vi "Format Target Name.vi"(8 "error in":errorcluster, 11 "OD Entry in":refnum<class "OD Entry.lvclass">) -> (0 "error out":errorcluster, 2 "Name":string, 3 "OD Entry out":refnum<class "OD Entry.lvclass">)   [LabVIEW 2019, in "PDO Grid.lvlib" / "PDO Mapping.lvclass"]
uses:
  PDO Mapping.lvclass
  Core/OD Entry/OD Entry.lvclass
  Core/OD Sub-Entry/OD Sub-Entry.lvclass
  D:/git/EDS-File-Viewer/source/Core/OD Entry/OD Entry.lvclass
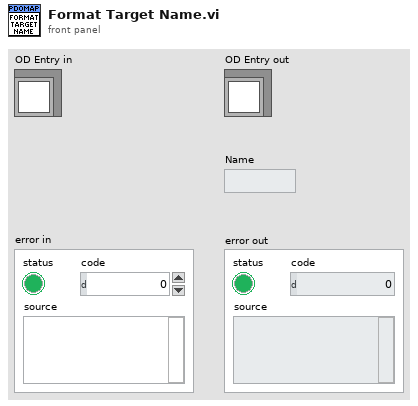
[diagram p1: front panel]
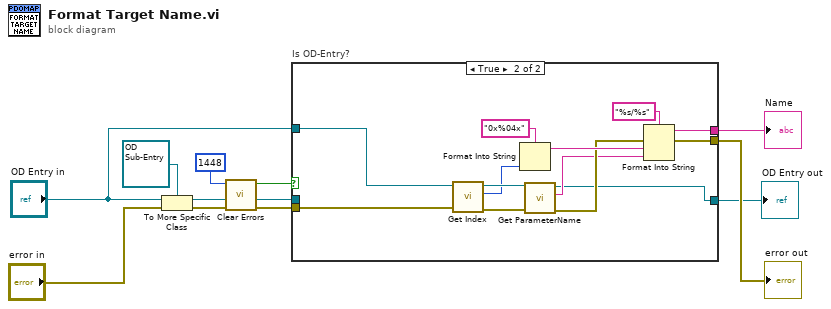
[diagram p0: block diagram]
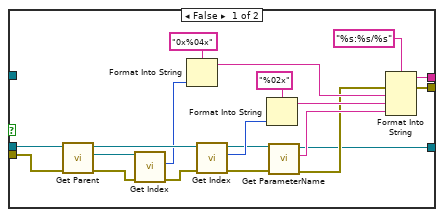
[diagram p2: hidden frame]
diagram:
  n1 = To More Specific Class(target class=refnum<class "OD Sub-Entry.lvclass"> refnum ("Electronic Datasheet.lvlib:OD Sub-Entry"), reference="OD Entry in", error in="error in") -> (specific class reference=w6:refnum<class "OD Sub-Entry.lvclass">, error out=w7:errorcluster)
  n2 = call <vilib>:"Clear Errors.vi"("error in (no error)"=w7, "specific error code to clear (0: all)"=1448) -> ("error out"=w4:errorcluster, "specific error cleared?"=w3:bool)  [unwired: 4 in]
  n3 = case "Is OD-Entry?" shown="True" w3 {
    tunnel: [w21 w33] -> w11
    tunnel: [w19 w35] -> w10
    tunnel: [w18 w34] -> w8
    tunnel: w6 -> [w12 _]
    tunnel: w4 -> [w17 w38]
    tunnel: "OD Entry in" -> [_ w32]
    frame False {
      n4 = call "Get Parent.vi"("Error In"=w17, "reference in"=w12) -> ("Error Out"=w16:errorcluster, "Parent"=w15:refnum<class "OD Entry.lvclass">, "reference out"=w31:refnum<class "OD Sub-Entry.lvclass">)  [unwired: 7 in]
      n5 = call "Get Index.vi"("Error In"=w16, "reference in"=w15) -> ("Error Out"=w30:errorcluster, "Index"=w13:u16)  [unwired: 7 in, 1 out]
      n6 = Format Into String(format string="0x%04x", w13) -> (resulting string=w24:string)  [unwired: 2 in, 1 out]
      n7 = call "Get Index.vi"("Error In"=w30, "reference in"=w31) -> ("Error Out"=w26:errorcluster, "Index"=w28:u16, "reference out"=w27:refnum<class "OD Sub-Entry.lvclass">)  [unwired: 7 in]
      n8 = Format Into String(format string="%02x", w28) -> (resulting string=w23:string)  [unwired: 2 in, 1 out]
      n9 = call "Get ParameterName.vi"("Error In"=w26, "reference in"=w27) -> ("Error Out"=w20:errorcluster, "ParameterName"=w22:string, "reference out"=w18:refnum<class "OD Sub-Entry.lvclass">)  [unwired: 7 in]
      n10 = Format Into String(format string="%s:%s/%s", error in=w20, w24, w23, w22) -> (resulting string=w21:string, error out=w19:errorcluster)  [unwired: 1 in]
    }
    frame True {
      n11 = call "Get Index.vi"("Error In"=w38, "reference in"=w32) -> ("Error Out"=w43:errorcluster, "Index"=w37:u16, "reference out"=w44:refnum<class "OD Entry.lvclass">)  [unwired: 7 in]
      n12 = Format Into String(format string="0x%04x", w37) -> (resulting string=w41:string)  [unwired: 2 in, 1 out]
      n13 = call "Get ParameterName.vi"("Error In"=w43, "reference in"=w44) -> ("Error Out"=w40:errorcluster, "ParameterName"=w36:string, "reference out"=w34:refnum<class "OD Entry.lvclass">)  [unwired: 7 in]
      n14 = Format Into String(format string="%s/%s", error in=w40, w41, w36) -> (resulting string=w33:string, error out=w35:errorcluster)  [unwired: 1 in]
    }
  }
  "Name" <- w11
  "error out" <- w10
  "OD Entry out" <- w8
